vi "Auto_Routine_Swerve2Piece.vi"(8 "error in (no error)":errorcluster) -> (0 "error out":errorcluster)   [LabVIEW 2023]
uses:
  Arm/ArmPositionPreset.ctl
  TrajectoryOrientation.ctl
  Arm/ArmGamePiecePreset.ctl
  <vilib>/Rock Robotics/WPI/ThirdParty/JAS_Junk/TrajLib/Trajectory_Library.lvlib
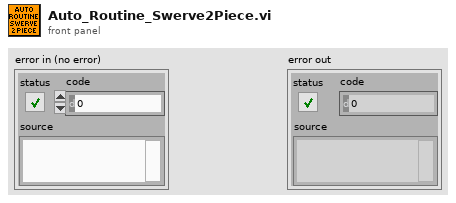
[diagram p1: front panel]
types:
  T1 = typedef "ArmGamePiecePreset.ctl" = enum16{"Cube", "Cone"}
  T2 = typedef "ArmPositionPreset.ctl" = enum16{"Upper", "Lower", "Middle", "Home", "Shelf", "Floor", "HalfFloor", "HalfHome"}
  T3 = typedef "TrajectoryOrientation.ctl" = enum16{"SameOrientation", "RotateToEndOrientation"}
  T4 = typedef "Trajectory_Library.lvlib/TRAJECTORY.ctl" = cluster{"TotalTImeSecs":dbl, "States":T5[]}
  T5 = typedef "Trajectory_Library.lvlib/TRAJ_STATE.ctl" = cluster{"TimeSeconds":dbl, "Velocity":dbl, "Acceleration":dbl, "POSE":T6, "Curvature":dbl}
  T6 = typedef "Trajectory_Library.lvlib/POSE2D.ctl" = cluster{"TRANSLATION":T7, "ROTATION":T8}
  T7 = typedef "Trajectory_Library.lvlib/TRANSLATION2D.ctl" = cluster{"X":dbl, "Y":dbl}
  T8 = typedef "Trajectory_Library.lvlib/ROTATION2D.ctl" = cluster{"VALUE":dbl, "COS":dbl, "SIN":dbl}
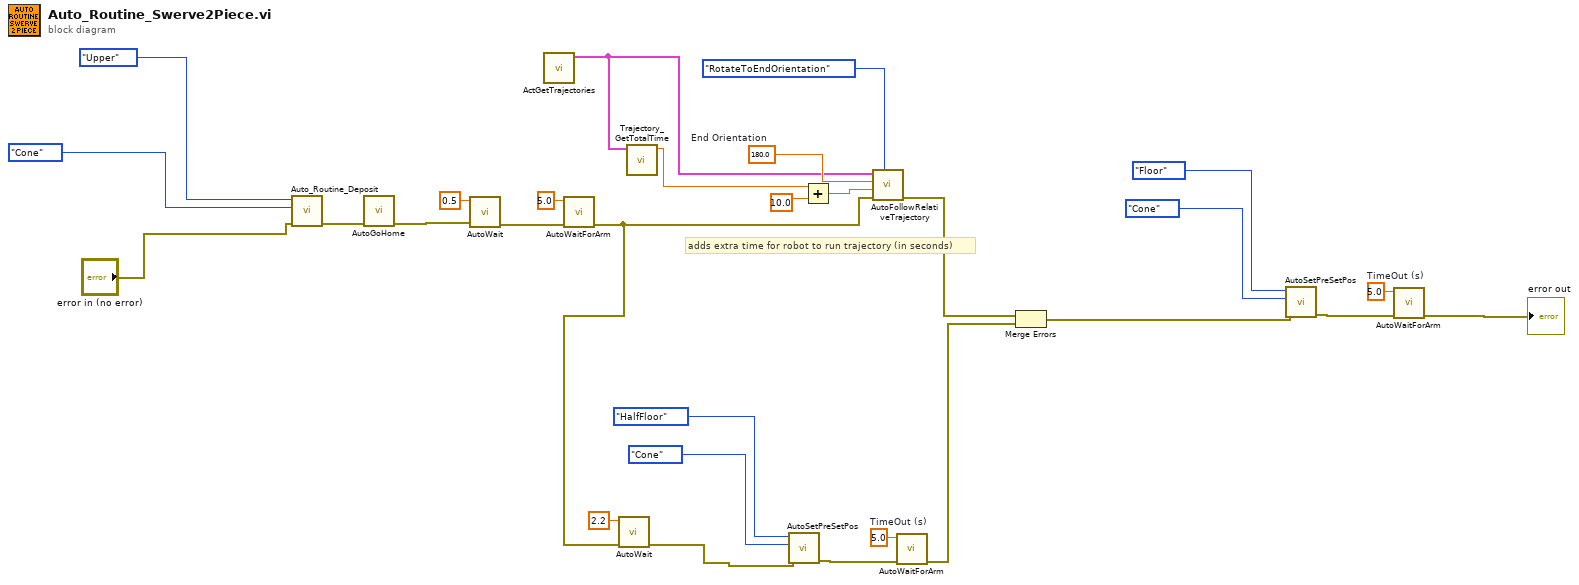
[diagram p0: block diagram]
diagram:
  w6 = 5.0  # TimeOut (s)
  w15 = 5.0  # TimeOut (s)
  w18 = 180.0  # End Orientation
  # "adds extra time for robot to run trajectory (in seconds)"
  n1 = call "Auto_Routine_Deposit.vi"("error in (no error)"="error in (no error)", "Game Piece"=ArmGamePiecePreset."Cone", "Position"=ArmPositionPreset."Upper") -> ("error out"=w22:errorcluster)  [unwired: 8 in]
  n2 = call "AutoGoHome.vi"("error in (no error)"=w22) -> ("error out"=w23:errorcluster)  [unwired: 10 in]
  n3 = call "AutoWait.vi"("error in (no error)"=w23, "TimeOut (s)"=0.5) -> ("error out"=w25:errorcluster)  [unwired: 9 in]
  n4 = call "ActGetTrajectories.vi"() -> ("Trajectory1"=w17:T4)  [unwired: 8 in, 3 out]
  n5 = call "AutoWaitForArm.vi"("error in (no error)"=w25, "TimeOut (s)"=5.0) -> ("error out"=w9:errorcluster)  [unwired: 9 in]
  n6 = call "AutoWait.vi"("error in (no error)"=w9, "TimeOut (s)"=2.2) -> ("error out"=w10:errorcluster)  [unwired: 9 in]
  n7 = call <vilib>:"Trajectory_GetTotalTime.vi"("TRAJECTORY"=w17) -> ("TotalTime_Sec"=w16:dbl)  [unwired: 10 in]
  n8 = call "AutoSetPreSetPos.vi"("error in (no error)"=w10, "Game Piece"=ArmGamePiecePreset."Cone", "Position"=ArmPositionPreset."HalfFloor") -> ("error out"=w13:errorcluster)  [unwired: 8 in]
  n9 = Add(x=w16, y=10.0) -> (x+y=w20:dbl)
  n10 = call "AutoFollowRelativeTrajectory.vi"("Orientation"=TrajectoryOrientation."RotateToEndOrientation", "error in (no error)"=w9, "TimeOut (s)"=w20, "End Orientation"=w18, "Trajectory"=w17) -> ("error out"=w8:errorcluster)  [unwired: 6 in]
  n11 = call "AutoWaitForArm.vi"("error in (no error)"=w13, "TimeOut (s)"=w15) -> ("error out"=w7:errorcluster)  [unwired: 9 in]
  n12 = Merge Errors(w8, w7) -> (w2:errorcluster)
  n13 = call "AutoSetPreSetPos.vi"("error in (no error)"=w2, "Game Piece"=ArmGamePiecePreset."Cone", "Position"=ArmPositionPreset."Floor") -> ("error out"=w4:errorcluster)  [unwired: 8 in]
  n14 = call "AutoWaitForArm.vi"("error in (no error)"=w4, "TimeOut (s)"=w6) -> ("error out"=→"error out":errorcluster)  [unwired: 9 in]
